vi "EventTest.vi"() -> ()   [LabVIEW 2019]
panel:
  out "OldVal":bool
  out "NewVal":bool
  out "Numeric":dbl
  in  "x > y?":bool
  out "Thermometer":dbl(slide) scale=0.0..100.0
  in  "stop 2":bool
  in  "Slide 2":dbl(slide) scale=0.0..10.0
  in  "Slide":dbl(slide) scale=0.0..10.0
  in  "stop":bool
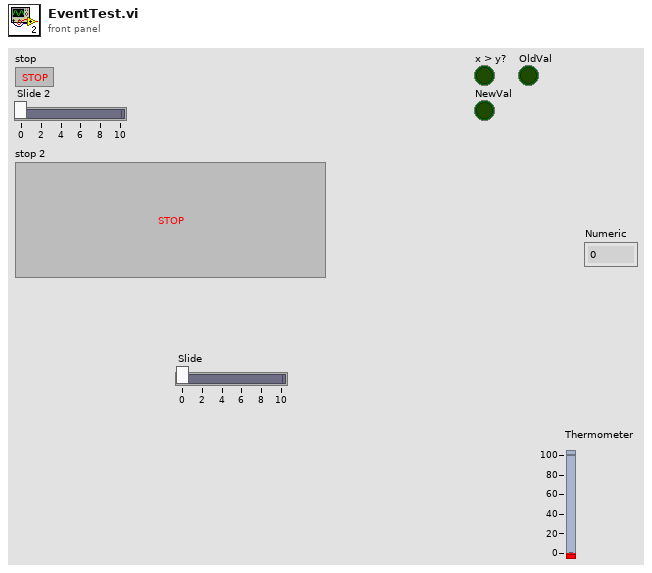
[diagram p1: front panel]
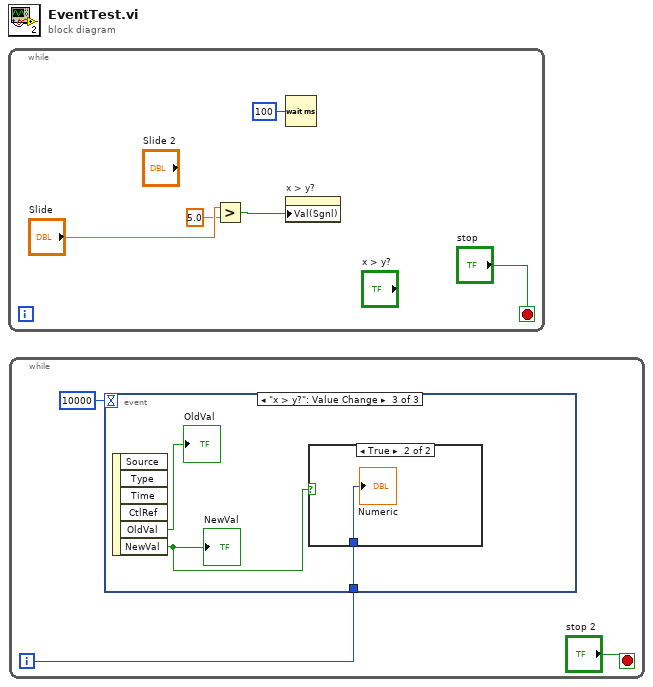
[diagram p0: block diagram]
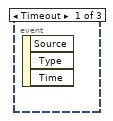
[diagram p2: hidden frame]
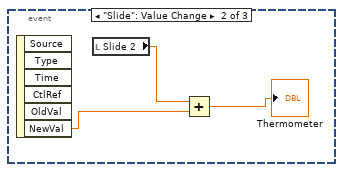
[diagram p3: hidden frame]
diagram:
  n1 = while {
    stop <- "stop" stop-if-true
    n2 = Greater?(x="Slide", y=5.0) -> (0:w1:bool)
    n3 = Wait (ms)(milliseconds to wait=u32 100) -> ()  [unwired: 1 out]
    n4 = property on="x > y?" class="Bool (strict)"("Val(Sgnl)"=w1) -> ()  [unwired: 2 in, 2 out]
  }
  n5 = while {
    i -> [w6]
    stop <- "stop 2" stop-if-true
    n6 = event shown="[2] \"x > y?\": Value Change" {
      selector: _ -> [_ _ _]
      dyn-events: _ -> [_ _ _]
      timeout: 10000 -> [_ _ _]
      tunnel: w6 -> [_ _ w14]
      event Timeout {
        n7 = event-data() -> ()  [unwired: 1 in, 3 out]
      }
      event "Slide": Value Change {
        n8 = event-data() -> ("NewVal"=w11:dbl)  [unwired: 1 in, 5 out]
        n9 = local read "Slide 2"() -> (w10:dbl)
        n10 = Add(x=w10, y=w11) -> (x+y=→"Thermometer":dbl)
      }
      event "x > y?": Value Change {
        n11 = event-data() -> ("OldVal"=→"OldVal":bool, "NewVal"=w12:bool)  [unwired: 1 in, 4 out]
        "NewVal" <- w12
        n12 = case shown="True" w12 {
          tunnel: w14 -> [_ w15]
          frame False {
          }
          frame True {
            "Numeric" <- w15
          }
        }
      }
    }
  }
